vi "tdms file.vi"(11 "String":string="hola") -> ()   [LabVIEW 2020, in "Logging.lvlib"]
uses:
  Logging.lvlib
  <vilib>/Utility/sysdir.llb/System Directory Type.ctl
  <vilib>/measure/NI_MABase.lvlib
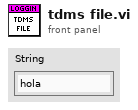
[diagram p1: front panel]
types:
  T1 = enum16{"Sine Wave", "Triangle Wave", "Square Wave", "Sawtooth Wave"}
  T2 = enum16{"open", "open or create", "create or replace", "create", "open (read-only)"}
  T3 = typedef "System Directory Type.ctl" = i32
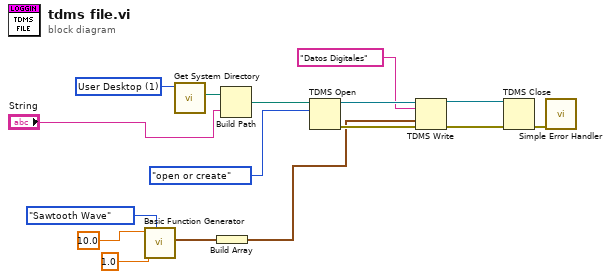
[diagram p0: block diagram]
diagram:
  w15 = T3 1 items=["User Home"=0, "User Desktop"=1, "User Documents"=2, "User Application Data"=3, "User Preferences"=4, "User Temporary"=5, "Public Documents"=6, "Public Application Data"=7, "Public Preferences"=8, "Public Cache"=13, "System Core Libraries"=9, "System Installed Libraries"=10, "Application Files"=11, "Boot Volume Root"=12] ("system directory type")
  n1 = call <vilib>:"Basic Function Generator.vi"("signal type"=T1."Sawtooth Wave", "amplitude"=1.0, "frequency"=10.0) -> ("signal out"=w6:waveform(dbl))  [unwired: 6 in, 2 out]
  n2 = call <vilib>:"Get System Directory.vi"("system directory type"=w15) -> ("system directory"=w14:path)  [unwired: 10 in]
  n3 = Build Array(w6) -> (w5:waveform(dbl)[])
  n4 = Build Path(base path=w14, name or relative path="String") -> (appended path=w16:path)
  n5 = TDMS Open(10:T2."open or create" ("operation (0:open)"), 11:w16) -> (0:w13:errorcluster, 3:w10:refnum<k34>)  [unwired: 5 in]
  n6 = TDMS Write(0:w10, 5:"Datos Digitales" ("group name in (Untitled)"), 9:w5, 11:w13) -> (4:w9:refnum<k34>, 15:w12:errorcluster)  [unwired: 2 in, 2 out]
  n7 = TDMS Close(8:w12, 11:w9) -> (0:w11:errorcluster)  [unwired: 1 out]
  n8 = call <vilib>:"Simple Error Handler.vi"("error in (no error)"=w11) -> ()  [unwired: 4 in, 5 out]
